vi "HDPE Erode and Dilate.vi"(8 "error in (no error)":errorcluster, 11 "Image Src":T1) -> (0 "error out":errorcluster, 3 "Image Dst Out":T1)   [LabVIEW 2019]
uses:
  <vilib>/vision/Image Controls.llb/IMAQ Image.ctl
  <vilib>/vision/NI_Vision_Development_Module.lvlib
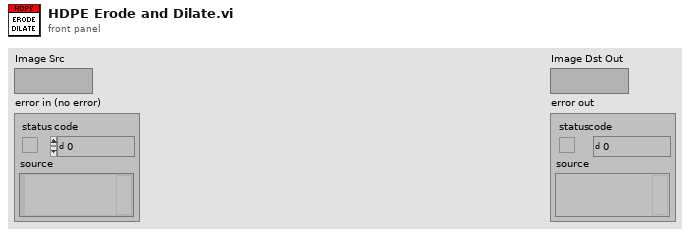
[diagram p1: front panel]
types:
  T1 = typedef "IMAQ Image.ctl" = refnum<image>
  T2 = enum32{"AutoM", "Close", "Dilate", "Erode", "Gradient", "Gradient out", "Gradient in", "Hit miss", "Open", "PClose", "POpen", "Thick", "Thin"}
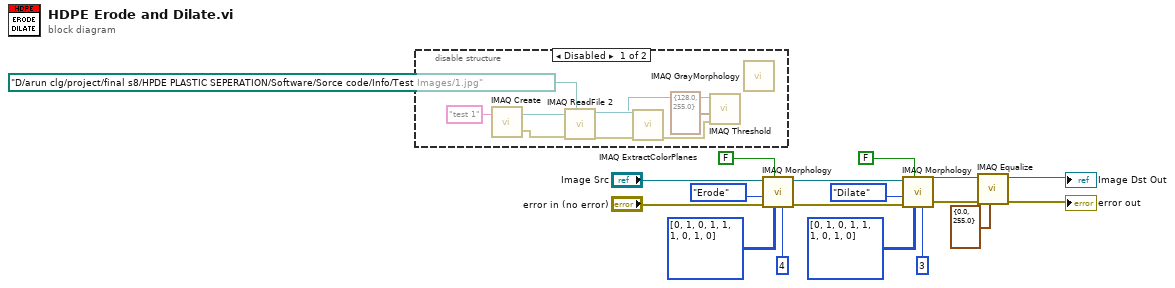
[diagram p0: block diagram]
diagram:
  n1 = disable-structure shown="Disabled" {
    frame Disabled {
      n2 = call "IMAQ Create"("Image Name"="test 1") -> ("New Image"=w26:T1, "error out"=w23:errorcluster)  [unwired: 4 in]
      n3 = call "IMAQ ReadFile 2"("File Path"=path "D:/arun clg/project/final s8/HPDE PLASTIC SEPERATION/Software/Sorce code/Info/Test Images/1.jpg", "error in (no error)"=w23, "Image"=w26) -> ("error out"=w21:errorcluster, "Image Out"=w22:T1)  [unwired: 4 in, 3 out]
      n4 = call "IMAQ ExtractColorPlanes"("error in (no error)"=w21, "Image Src"=w22) -> ("error out"=w19:errorcluster, "Red or Hue Plane out"=w20:T1)  [unwired: 6 in, 2 out]
      n5 = call "IMAQ Threshold"("error in (no error)"=w19, "Range"=cluster{"Lower value":sgl, "Upper value":sgl} {"Lower value"=128.0, "Upper value"=255.0}, "Image Src"=w20) -> ()  [unwired: 7 in, 2 out]
      n6 = call "IMAQ GrayMorphology"() -> ()  [unwired: 10 in, 2 out]
    }
    frame Enabled {
    }
  }
  n7 = call "IMAQ Morphology"("Number of iterations (1)"=4, "Structuring Element"=i32[][] [[0, 1, 0], [1, 1, 1], [0, 1, 0]], "Square/Hexa (Square)"=FALSE, "error in (no error)"="error in (no error)", "Operation"=T2."Erode", "Image Src"="Image Src") -> ("error out"=w12:errorcluster, "Image Dst Out"=w17:T1)  [unwired: 1 in, 3 out]
  n8 = call "IMAQ Morphology"("Number of iterations (1)"=3, "Structuring Element"=i32[][] [[0, 1, 0], [1, 1, 1], [0, 1, 0]], "Square/Hexa (Square)"=FALSE, "error in (no error)"=w12, "Operation"=T2."Dilate", "Image Src"=w17) -> ("error out"=w3:errorcluster, "Image Dst Out"=w5:T1)  [unwired: 1 in, 3 out]
  n9 = call "IMAQ Equalize"("Range"=cluster{"Minimum":sgl, "Maximum":sgl} {"Minimum"=0.0, "Maximum"=255.0}, "error in (no error)"=w3, "Image Src"=w5) -> ("error out"=→"error out":errorcluster, "Image Dst Out"=→"Image Dst Out":T1)  [unwired: 3 in, 4 out]
